vi "E Series Reader.vi"(8 "error in":errorcluster, 11 "File name":string[](array[string])) -> (0 "error out":errorcluster, 3 "E Series":T1)   [LabVIEW 2018, in "E Series Reader.lvlib"]
uses:
  E Series Reader.lvlib
  Data--control.ctl
  States--control.ctl
  Index--control.ctl
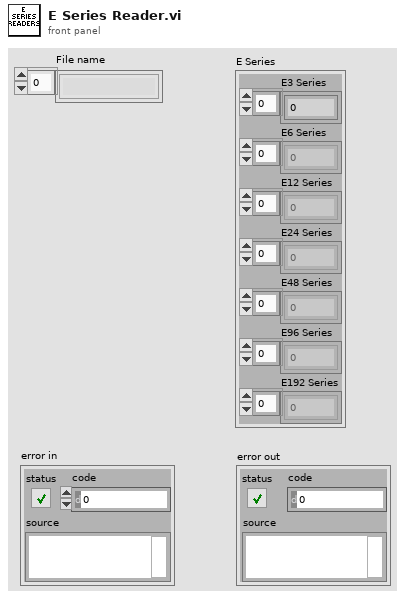
[diagram p1: front panel]
types:
  T1 = typedef "E Series Reader.lvlib/Data--control.ctl" = cluster{"E3 Series":u16[], "E6 Series ":u16[], "E12 Series":u16[], "E24 Series":u16[], "E48 Series":u16[], "E96 Series":u16[], "E192 Series":u16[]}
  T2 = typedef "E Series Reader.lvlib/States--control.ctl" = enum16{"Initialize", "Read E3", "Read E6", "Read E12", "Read E24", "Read E48", "Read E96", "Read E192", "Error", "Shutdown"}
  T3 = typedef "E Series Reader.lvlib/Index--control.ctl" = enum16{"E3", "E6", "E12", "E24", "E48", "E96", "E192"}
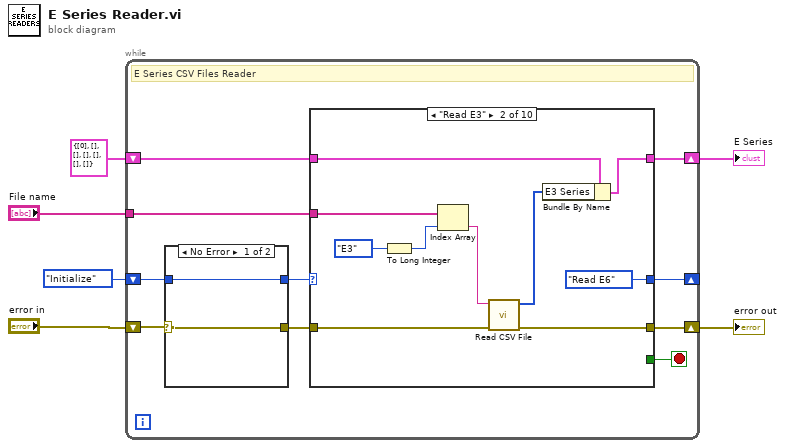
[diagram p0: block diagram]
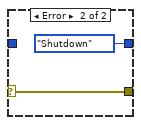
[diagram p2: hidden frame]
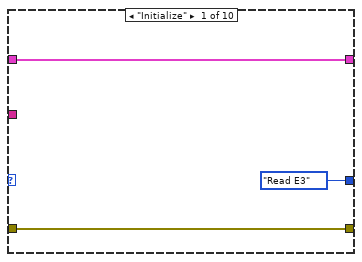
[diagram p3: hidden frame]
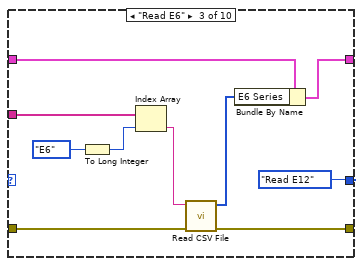
[diagram p4: hidden frame]
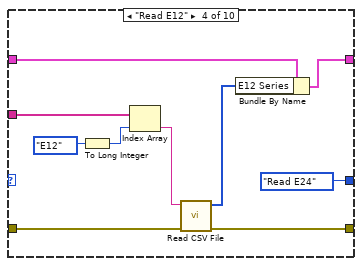
[diagram p5: hidden frame]
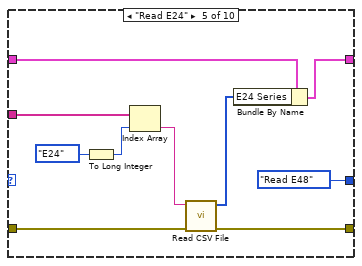
[diagram p6: hidden frame]
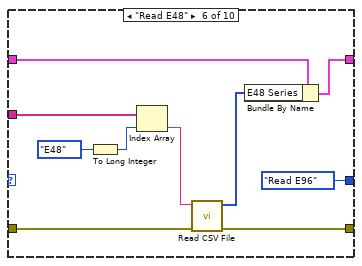
[diagram p7: hidden frame]
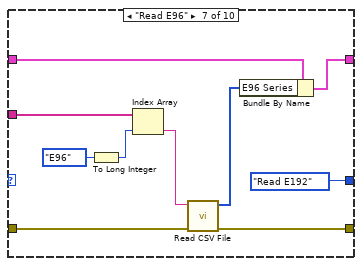
[diagram p8: hidden frame]
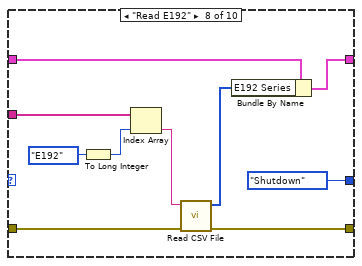
[diagram p9: hidden frame]
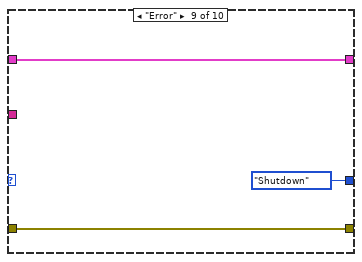
[diagram p10: hidden frame]
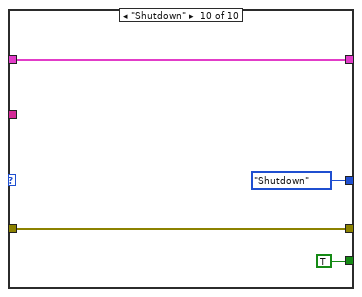
[diagram p11: hidden frame]
diagram:
  n1 = while {
    shift-right: [w11] -> _
    shift-left: States--control."Initialize" -> [w16]
    shift-right: [w13] -> w5
    shift-left: "error in" -> [w15]
    shift-right: [w8] -> w1
    shift-left: T1 {"E3 Series"=[0], "E6 Series "=[], "E12 Series"=[], "E24 Series"=[], "E48 Series"=[], "E96 Series"=[], "E192 Series"=[]} -> [w9]
    tunnel: "File name" -> [w7]
    stop <- w10 stop-if-true
    # "E Series CSV Files Reader"
    n2 = case shown="No Error" w15 {
      selector: w15 -> [w18 w20]
      tunnel: w16 -> [w17 _]
      tunnel: [w18 w20] -> w14
      tunnel: [w17 States--control."Shutdown"] -> w12
      frame No Error {
      }
      frame Error {
      }
    }
    n3 = case shown="\"Read E3\"" w12 {
      tunnel: w14 -> [w23 w29 w39 w52 w62 w72 w82 w89 w96 w99]
      tunnel: [w23 w28 w40 w51 w61 w71 w81 w88 w96 w99] -> w13
      tunnel: [States--control."Read E3" States--control."Read E6" States--control."Read E12" States--control."Read E24" States--control."Read E48" States--control."Read E96" States--control."Read E192" States--control."Shutdown" States--control."Shutdown" States--control."Shutdown"] -> w11
      tunnel: [_ _ _ _ _ _ _ _ _ TRUE] -> w10
      tunnel: w9 -> [w21 w32 w42 w50 w60 w70 w80 w92 w94 w97]
      tunnel: [w21 w31 w41 w48 w59 w69 w79 w91 w94 w97] -> w8
      tunnel: w7 -> [_ w27 w35 w45 w55 w64 w75 w85 _ _]
      frame "Initialize" {
      }
      frame "Read E3" {
        n4 = To Long Integer(number=Index--control."E3") -> (32bit integer=w24:i32)
        n5 = Index Array(array=w27, index=w24) -> (element=w26:string)
        n6 = call "Read CSV File.vi"("error in (no error)"=w29, "Serie File Name"=w26) -> ("error out"=w28:errorcluster, "Serie"=w30:u16[])  [unwired: 8 in]
        n7 = Bundle By Name(cluster=w32, "E3 Series"=w30) -> (w31:T1)
      }
      frame "Read E6" {
        n8 = To Long Integer(number=Index--control."E6") -> (32bit integer=w36:i32)
        n9 = Index Array(array=w35, index=w36) -> (element=w34:string)
        n10 = call "Read CSV File.vi"("error in (no error)"=w39, "Serie File Name"=w34) -> ("error out"=w40:errorcluster, "Serie"=w38:u16[])  [unwired: 8 in]
        n11 = Bundle By Name(cluster=w42, "E6 Series"=w38) -> (w41:T1)
      }
      frame "Read E12" {
        n12 = To Long Integer(number=Index--control."E12") -> (32bit integer=w47:i32)
        n13 = Index Array(array=w45, index=w47) -> (element=w44:string)
        n14 = call "Read CSV File.vi"("error in (no error)"=w52, "Serie File Name"=w44) -> ("error out"=w51:errorcluster, "Serie"=w49:u16[])  [unwired: 8 in]
        n15 = Bundle By Name(cluster=w50, "E12 Series"=w49) -> (w48:T1)
      }
      frame "Read E24" {
        n16 = To Long Integer(number=Index--control."E24") -> (32bit integer=w57:i32)
        n17 = Index Array(array=w55, index=w57) -> (element=w54:string)
        n18 = call "Read CSV File.vi"("error in (no error)"=w62, "Serie File Name"=w54) -> ("error out"=w61:errorcluster, "Serie"=w58:u16[])  [unwired: 8 in]
        n19 = Bundle By Name(cluster=w60, "E24 Series"=w58) -> (w59:T1)
      }
      frame "Read E48" {
        n20 = To Long Integer(number=Index--control."E48") -> (32bit integer=w67:i32)
        n21 = Index Array(array=w64, index=w67) -> (element=w65:string)
        n22 = call "Read CSV File.vi"("error in (no error)"=w72, "Serie File Name"=w65) -> ("error out"=w71:errorcluster, "Serie"=w68:u16[])  [unwired: 8 in]
        n23 = Bundle By Name(cluster=w70, "E48 Series"=w68) -> (w69:T1)
      }
      frame "Read E96" {
        n24 = To Long Integer(number=Index--control."E96") -> (32bit integer=w77:i32)
        n25 = Index Array(array=w75, index=w77) -> (element=w74:string)
        n26 = call "Read CSV File.vi"("error in (no error)"=w82, "Serie File Name"=w74) -> ("error out"=w81:errorcluster, "Serie"=w78:u16[])  [unwired: 8 in]
        n27 = Bundle By Name(cluster=w80, "E96 Series"=w78) -> (w79:T1)
      }
      frame "Read E192" {
        n28 = To Long Integer(number=Index--control."E192") -> (32bit integer=w87:i32)
        n29 = Index Array(array=w85, index=w87) -> (element=w84:string)
        n30 = call "Read CSV File.vi"("error in (no error)"=w89, "Serie File Name"=w84) -> ("error out"=w88:errorcluster, "Serie"=w90:u16[])  [unwired: 8 in]
        n31 = Bundle By Name(cluster=w92, "E192 Series"=w90) -> (w91:T1)
      }
      frame "Error" {
      }
      frame "Shutdown" {
      }
    }
  }
  "error out" <- w5
  "E Series" <- w1
